vi "NI Switch Debounced.vi"(8 "error in (no error)":errorcluster, 11 "RelayOutput in":refnum<class "NISwitch.lvclass">) -> (0 "error out":errorcluster, 2 "is debounced":bool, 3 "RelayOutput out":refnum<class "NISwitch.lvclass">)   [LabVIEW 2023, in "HardwareAbstractionLayer_LVOOP.lvlib" / "NISwitch.lvclass"]
uses:
  NISwitch.lvclass
  NISwitch.lvclass/NISwitch.ctl
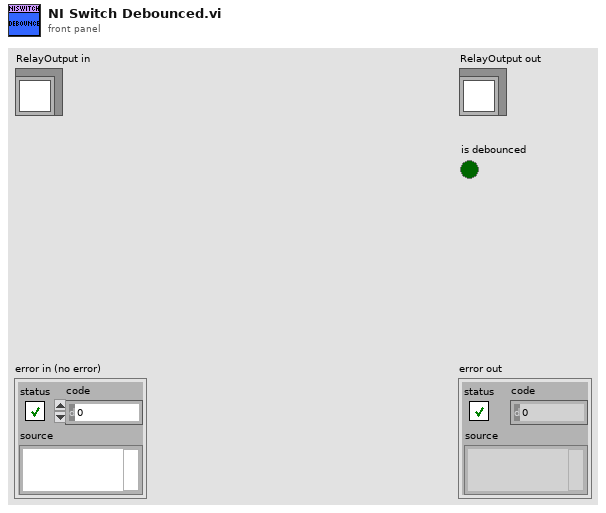
[diagram p1: front panel]
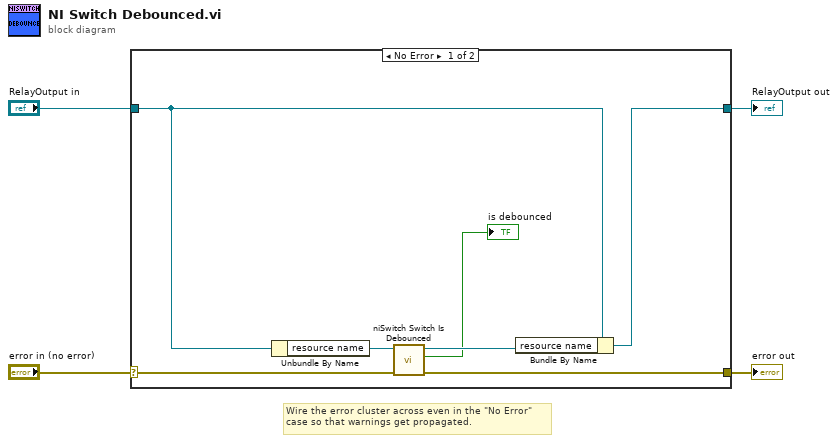
[diagram p0: block diagram]
diagram:
  # "Wire the error cluster across even in the \"No Error\"\ncase so that warnings get propagated."
  n1 = case shown="No Error" "error in (no error)" {
    selector: "error in (no error)" -> [w11 w13]
    tunnel: [w10 w13] -> w3
    tunnel: [w7 w12] -> w1
    tunnel: "RelayOutput in" -> [w8 w12]
    frame No Error {
      n2 = Unbundle By Name(w8) -> ("resource name"=w9:refnum<k15>)
      n3 = call <instrlib>:"niSwitch Switch Is Debounced.vi"("error in (no error)"=w11, "instrument handle"=w9) -> ("error out"=w10:errorcluster, "is debounced"=→"is debounced":bool, "instrument handle out"=w6:refnum<k15>)  [unwired: 7 in]
      n4 = Bundle By Name(cluster=w8, "resource name"=w6) -> (w7:refnum<class "NISwitch.lvclass">)
    }
    frame Error {
    }
  }
  "error out" <- w3
  "RelayOutput out" <- w1
